vi "AlliGator Fit IRF String.vi"(8 "Error In":errorcluster, 9 "IRF":T1, 11 "Use Local IRF":bool) -> (0 "Error Out":errorcluster, 1 "IRF String":string)   [LabVIEW 2021, in "AlliGator Decay Analysis.lvlib" / "AlliGator Decay Fit.lvlib"]
doc: "Create the Notebook string specifying what kind of IRF was used in the fit."
uses:
  Graphs/XY Graph/XY Plot Data.ctl
  AlliGator Decay Fit.lvlib
  Graphs/XY Graph/XY Graph Add-Ons.lvlib
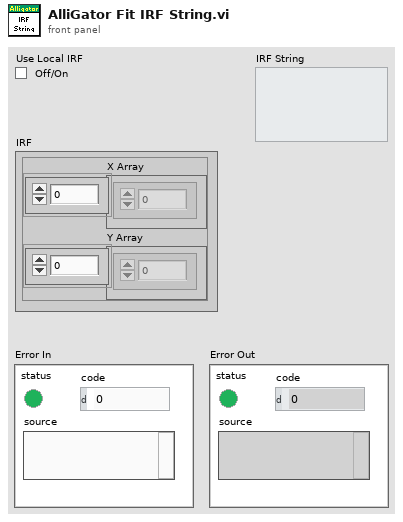
[diagram p1: front panel]
types:
  T1 = typedef "XY Graph Add-Ons.lvlib/XY Plot Data.ctl" = cluster{"X Array":dbl[], "Y Array":dbl[]}
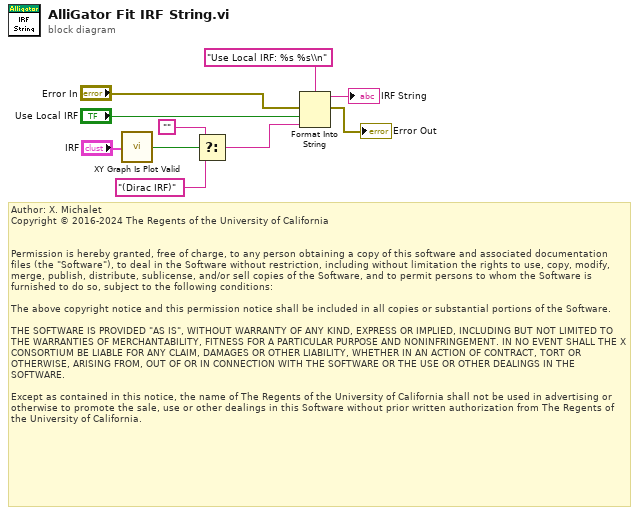
[diagram p0: block diagram]
diagram:
  # "Author: X. Michalet\nCopyright © 2016-2024 The Regents of the University of California\n \n\nPermission is hereby granted, free of charge, to any person obtaining a copy of this software and associated documentation files (the \"Software\"), to deal in the Software without restriction, including without limitation the rights to use, copy, modify, merge, publish, distribute, sublicense, and/or sell copies of the Software, and to permit persons to whom the Software is furnished to do so, subject to the following conditions:\n\nThe above copyright notice and this permission notice shall be included in all copies or substantial portions of the Software.\n\nTHE SOFTWARE IS PROVIDED \"AS IS\", WITHOUT WARRANTY OF ANY KIND, EXPRESS OR IMPLIED, INCLUDING BUT NOT LIMITED TO THE WARRANTIES OF MERCHANTABILITY, FITNESS FOR A PARTICULAR PURPOSE AND NONINFRINGEMENT. IN NO EVENT SHALL THE X CONSORTIUM BE LIABLE FOR ANY CLAIM, DAMAGES OR OTHER LIABILITY, WHETHER IN AN ACTION OF CONTRACT, TORT OR OTHERWISE, ARISING FROM, OUT OF OR IN CONNECTION WITH THE SOFTWARE OR THE USE OR OTHER DEALINGS IN THE SOFTWARE.\n\nExcept as contained in this notice, the name of The Regents of the University of California shall not be used in advertising or otherwise to promote the sale, use or other dealings in this Software without prior written authorization from The Regents of the University of California."
  n1 = call "XY Graph Is Plot Valid.vi"("Plot"="IRF") -> ("Is Valid Plot?"=w6:bool)  [unwired: 8 in]
  n2 = Select(t="", s=w6, f="(Dirac IRF)") -> (s? t:f=w3:string)
  n3 = Format Into String(format string="Use Local IRF: %s %s\\n", error in="Error In", "Use Local IRF", w3) -> (resulting string=→"IRF String":string, error out=→"Error Out":errorcluster)  [unwired: 1 in]
